vi "DrawGaxes.vi"(1 "Shape":cluster{"length":sgl, "width/height":sgl}, 2 "world in":refnum<vi>) -> (0 "world out":refnum<vi>)   [LabVIEW 2012]
uses:
  <vilib>/picture/3D Picture Control/NI_3D Picture Control.lvlib
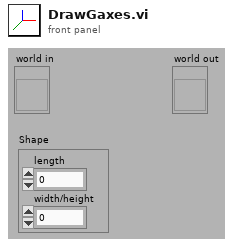
[diagram p1: front panel]
types:
  T1 = cluster{"Red":sgl, "Green":sgl, "Blue":sgl, "Alpha":sgl}
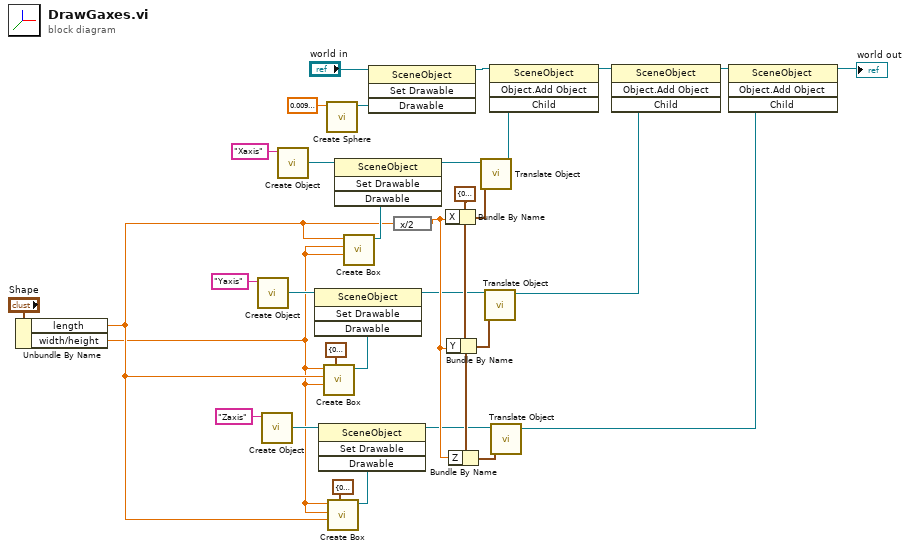
[diagram p0: block diagram]
diagram:
  w31 = cluster{"X":sgl, "Y":sgl, "Z":sgl} {"X"=0.0, "Y"=0.0, "Z"=0.0} ("Translation")
  n1 = Unbundle By Name("Shape") -> ("length"=w2:sgl, "width/height"=w1:sgl)
  n2 = call <vilib>:"Create Object.vi"("Name"="Yaxis") -> ("Scene:New Object"=w13:refnum<vi>)  [unwired: 1 in, 9 out]
  n3 = call <vilib>:"Create Object.vi"("Name"="Zaxis") -> ("Scene:New Object"=w26:refnum<vi>)  [unwired: 1 in, 9 out]
  n4 = call <vilib>:"Create Object.vi"("Name"="Xaxis") -> ("Scene:New Object"=w9:refnum<vi>)  [unwired: 1 in, 9 out]
  n5 = call <vilib>:"Create Box.vi"("Color"=T1 {"Red"=0.0, "Green"=1.0, "Blue"=0.0, "Alpha"=1.0}, "Length Z"=w1, "Length Y"=w2, "Length X"=w1) -> ("New Box Refnum"=w15:refnum<vi>)  [unwired: 6 in, 1 out]
  n6 = invoke class="SceneObject" method="Set Drawable"(reference=w13, "Drawable"=w15) -> (reference out=w19:refnum<vi>)  [unwired: 2 in, 3 out]
  n7 = call <vilib>:"Create Sphere.vi"("Radius"=sgl 0.01) -> ("New Sphere Refnum"=w6:refnum<vi>)  [unwired: 9 in, 1 out]
  n8 = call <vilib>:"Create Box.vi"("Color"=T1 {"Red"=0.0, "Green"=0.0, "Blue"=1.0, "Alpha"=1.0}, "Length Z"=w2, "Length Y"=w1, "Length X"=w1) -> ("New Box Refnum"=w24:refnum<vi>)  [unwired: 6 in, 1 out]
  n9 = invoke class="SceneObject" method="Set Drawable"(reference=w26, "Drawable"=w24) -> (reference out=w23:refnum<vi>)  [unwired: 2 in, 3 out]
  n10 = call <vilib>:"Create Box.vi"("Length Z"=w1, "Length Y"=w1, "Length X"=w2) -> ("New Box Refnum"=w7:refnum<vi>)  [unwired: 7 in, 1 out]
  n11 = invoke class="SceneObject" method="Set Drawable"(reference=w9, "Drawable"=w7) -> (reference out=w17:refnum<vi>)  [unwired: 2 in, 3 out]
  n12 = invoke class="SceneObject" method="Set Drawable"(reference="world in", "Drawable"=w6) -> (reference out=w10:refnum<vi>)  [unwired: 2 in, 3 out]
  n13 = expression code="x/2"(w2) -> (w32:sgl)
  n14 = Bundle By Name(cluster=w31, "X"=w32) -> (w11:cluster{"X":sgl, "Y":sgl, "Z":sgl})
  n15 = Bundle By Name(cluster=w31, "Y"=w32) -> (w12:cluster{"X":sgl, "Y":sgl, "Z":sgl})
  n16 = Bundle By Name(cluster=w31, "Z"=w32) -> (w27:cluster{"X":sgl, "Y":sgl, "Z":sgl})
  n17 = call <vilib>:"Translate Object.vi"("Translation"=w11, "Scene.Object In"=w17) -> ("Scene.Object Out"=w18:refnum<vi>)  [unwired: 8 in, 1 out]
  n18 = call <vilib>:"Translate Object.vi"("Translation"=w12, "Scene.Object In"=w19) -> ("Scene.Object Out"=w20:refnum<vi>)  [unwired: 8 in, 1 out]
  n19 = invoke class="SceneObject" method="Object.Add Object"(reference=w10, "Child"=w18) -> (reference out=w16:refnum<vi>)  [unwired: 2 in, 3 out]
  n20 = call <vilib>:"Translate Object.vi"("Translation"=w27, "Scene.Object In"=w23) -> ("Scene.Object Out"=w30:refnum<vi>)  [unwired: 8 in, 1 out]
  n21 = invoke class="SceneObject" method="Object.Add Object"(reference=w16, "Child"=w20) -> (reference out=w28:refnum<vi>)  [unwired: 2 in, 3 out]
  n22 = invoke class="SceneObject" method="Object.Add Object"(reference=w28, "Child"=w30) -> (reference out=→"world out":refnum<vi>)  [unwired: 2 in, 3 out]
